vi "TestHarnessDPL-DetBoardOnly-DESKTOP-REOD41B.vi"() -> ()   [LabVIEW 2025]
uses:
  <vilib>/Analysis/6fits.llb/Curve Fitting Criteria.ctl
  <vilib>/Analysis/1siggen.llb/Ramp Pattern by Samples.vi
  <vilib>/Analysis/1siggen.llb/Ramp Pattern by Delta.vi
  <vilib>/Analysis/NI_AALBase.lvlib
  <userlib>/_OpenG.lib/time/time.llb/openg_time.lvlib
  instr.lib/Detector SCPI/Detector SCPI.lvlib
  instr.lib/Keithley 24XX/Keithley 24XX.lvlib
  instr.lib/Keithley 648X Series/Keithley 648X Series.lvlib
  <vilib>/Analysis/NI_AALPro.lvlib
panel:
  out "error out":errorcluster
  out "OpVsCurrent":cluster{"Ramp Pattern":dbl[], dbl[]}[](array[cluster])
  in  "Exit":bool
  in  "Measurement Mode":T1(tab)
  in  "DetectorData":T2(array[cluster]) {"DAC Offset" min=1 max=4095 step=1}
  in  "SPI Clock":i64=1000000
  in  "Oversample":i32=1 min=1 max=4096
  in  "Power":bool=TRUE
  in  "Detector VISA":refnum<visa-resource-name>="Detector_EGSE"
  out "Detector Resource":refnum<visa-resource-name>="COM4"
  out "Voltage (V)":dbl[](array[numeric])=[3.264, 0.0, 12.488, 12.77]
  out "Current (mA)":dbl[](array[numeric])=[0.0, 0.0, 21.6, -3.65]
  in  "ThrowAway":i32=100 min=1 max=10000
  out "Detector EGSE ID String":string="Aberystwyth University,Enfys Detector,#01,v0.5.0\r\n"
  in  "Current source":refnum<visa-resource-name>
  in  "Channel":i32 min=0 max=7
  in  "Collection":enum16{"Science", "Debug"}(ring)
  in  "Tolerance":dbl
  in  "Target Counts":i32 min=0 max=4095
  in  "Find Offset":bool
  out "Searching...":bool
  out "BoardTemperature":dbl
  in  "Tab Control":enum32{"Counts", "All Counts", "Temperature"}(tab)
  out "Counts":dbl(graph)=160.194
  out "All Counts":T3(graph)
  out "Temperature":dbl(graph)=160.194
  in  "ResetVDACstats":bool
  in  "Gain":u16(ring) items=["High", "Med", "Low"]
  in  "DAC Value":i32=2076 min=0 max=4095 step=1
  in  "Detector":u16(ring) items=["SWIR", "MWIR"]
  out "Peak-to-Peak (counts)":dbl=0.0026870000001508743 format="%^.4g"
  out "rms (counts) 2":dbl=-2.7284841053187847e-12 format="%^.4g"
  out "Mean Value (counts)":dbl
  out "Elapsed(uS)":i32
  out "size":i32
  in  "Pause":bool
  out "XY Graph":cluster{dbl[], "subarray":dbl[]}(graph)
  in  "Detector 3":u16(ring) items=["SWIR", "MWIR"]
  in  "Gain 3":u16(ring) items=["High", "Med", "Low"]
  in  "trig":dbl=8.0 min=0.0 max=50.0
  in  "DetectorDAC":i32=2076 min=0 max=4095 step=1
  in  "Abort":bool
  out "Output vs current":cluster{"Ramp Pattern":dbl[], dbl[]}[](graph)
  in  "ISweep":bool
  in  "NPoints":i32=10 min=10 max=10000 step=1
  in  "MaxCurrent":dbl=1e-11 min=1e-11 max=1e-06
  in  "MinCurrent":dbl=1e-12 min=-10.0 max=10.0
  in  "Detector 4":u16(ring) items=["SWIR", "MWIR"]
  in  "LogSweep":bool
  in  "Gain 4":u16(ring) items=["High", "Med", "Low"]
  out "slope (counts/nA)":dbl
  out "intercept":dbl
  out "residue":dbl
  out "Max Deviation (counts)":dbl
  in  "DAC":i32 min=0 max=4095 step=1
  in  "Modulation Steps":i32=2 min=2 max=1000 step=1
  in  "Modulation Max":dbl min=0.0 max=10.0
  in  "Modulation Min":dbl min=-10.0 max=10.0
  in  "SweepLight":bool
  in  "Detector 7":u16(ring) items=["SWIR", "MWIR"]
  out "Output vs Light":cluster{dbl[], dbl[]}[](graph)
  in  "Gain 2":u16(ring) items=["High", "Med", "Low"]
  in  "Abort 2":bool
  in  "SweepVDAC":bool
  in  "ISource":dbl min=-1e-06 max=1e-06
  in  "VDAC Step":i32=1 min=1 max=100
  in  "VDAC Max":i32 min=0 max=4095
  in  "VDAC Min":i32 min=0 max=4000
  in  "Detector 5":u16(ring) items=["SWIR", "MWIR"]
  out "VDAC Sweep":cluster{dbl[], dbl[]}[](graph)
  in  "Abort SweepVDAC":bool
  in  "Step":bool
  in  "Delay 1 (ms)":i32
  in  "Current 2":dbl
  in  "Current 1":dbl
  out "Step Response":cluster{dbl[], "subarray":dbl[]}(graph)
  in  "chan (0)":i32
  out "exit":bool=TRUE
  # "3.3V supply"
  # "Heater"
  # "+12V Supply"
  # "-12V Supply"
  # "Pause button will halt collection and display.\nThis allows graph to be printed etc."
  # "Burst mode is intended to examine behaviour of the ADC\n\nA burst of readings is recorded on the EGSE and then gathered here."
  # "Light source modulated by USB205L working as voltage source connected to MOD input of LD250C\nreference photodiode monitored by 6846 picoammeter"
  # "Set current to Current#1. Waits for Delay 1 to stabilise, then switches to current 2 and reads 1000 readings as fast as possible"
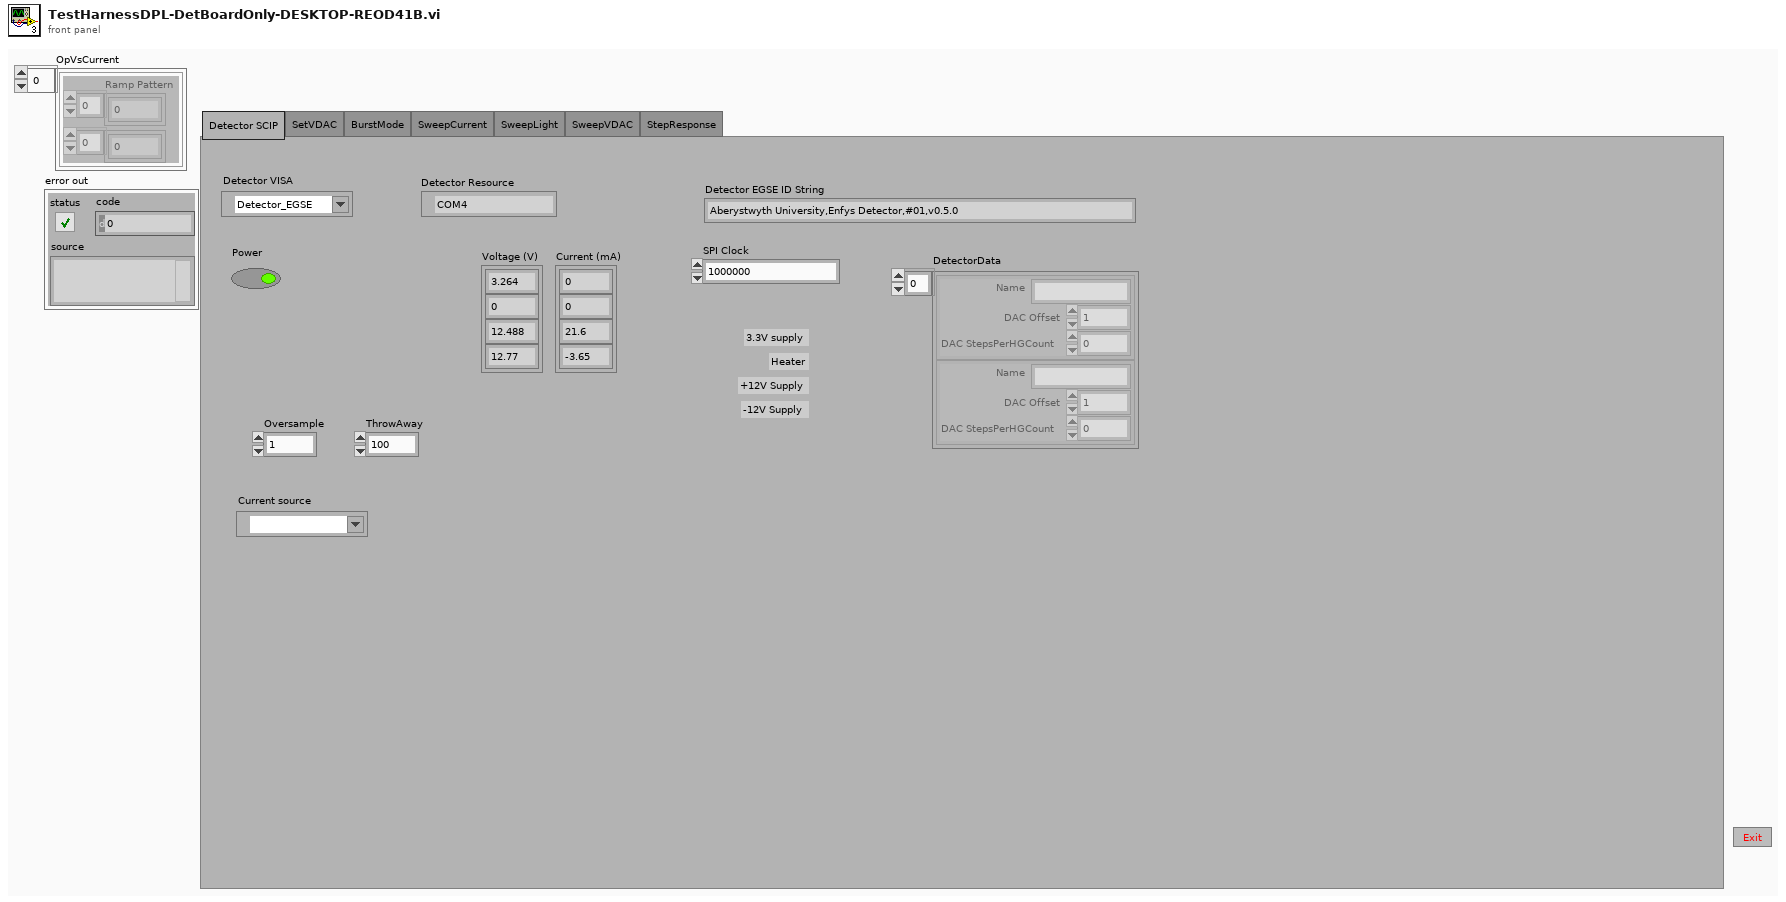
[diagram p1: front panel]
types:
  T1 = enum32{"Detector SCIP", "SetVDAC", "BurstMode", "SweepCurrent", "SweepLight", "SweepVDAC", "StepResponse"}
  T2 = cluster{"Name":string, "DAC Offset":i32, "DAC StepsPerHGCount":dbl}[]
  T3 = cluster{"subarray[0]":dbl, "subarray[1]":dbl, "subarray[2]":dbl, "subarray[3]":dbl, "subarray[4]":dbl, "subarray[5]":dbl, "subarray[6]":dbl, "subarray[7]":dbl, "subarray[8]":dbl}
  T4 = cluster{"Baud Rate":u32, "Parity":u16, "Data Bits":u16, "Stop Bits":u16, "Flow Control":u16}
  T5 = cluster{"Name":string, "DAC Offset":i32, "DAC StepsPerHGCount":dbl}
  T6 = typedef "NI_AALPro.lvlib/Curve Fitting Criteria.ctl" = u16
  T7 = typedef "LVPointDoubleTypeDef.ctl" = cluster{"Cursor X":dbl, "Cursor Y":dbl}
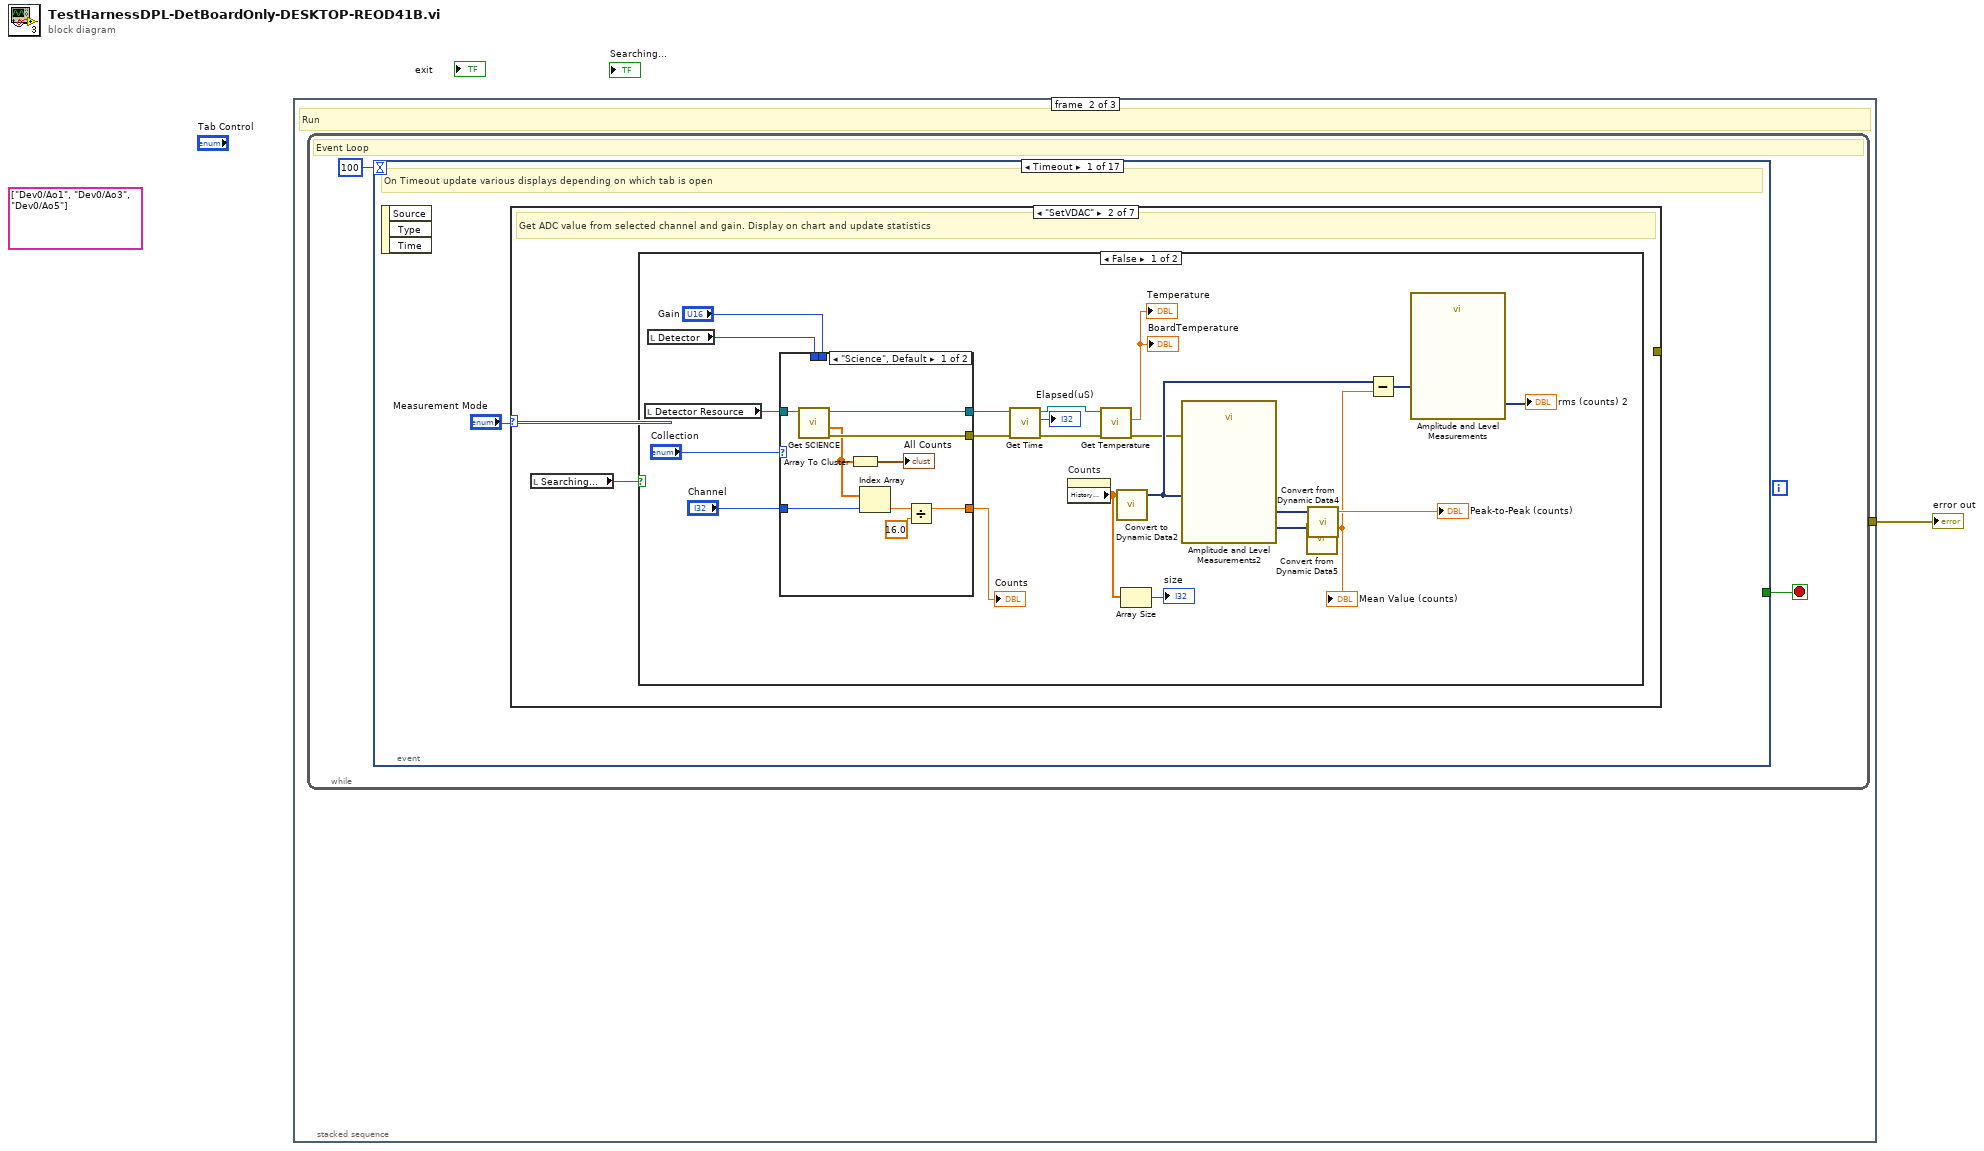
[diagram p0: block diagram]
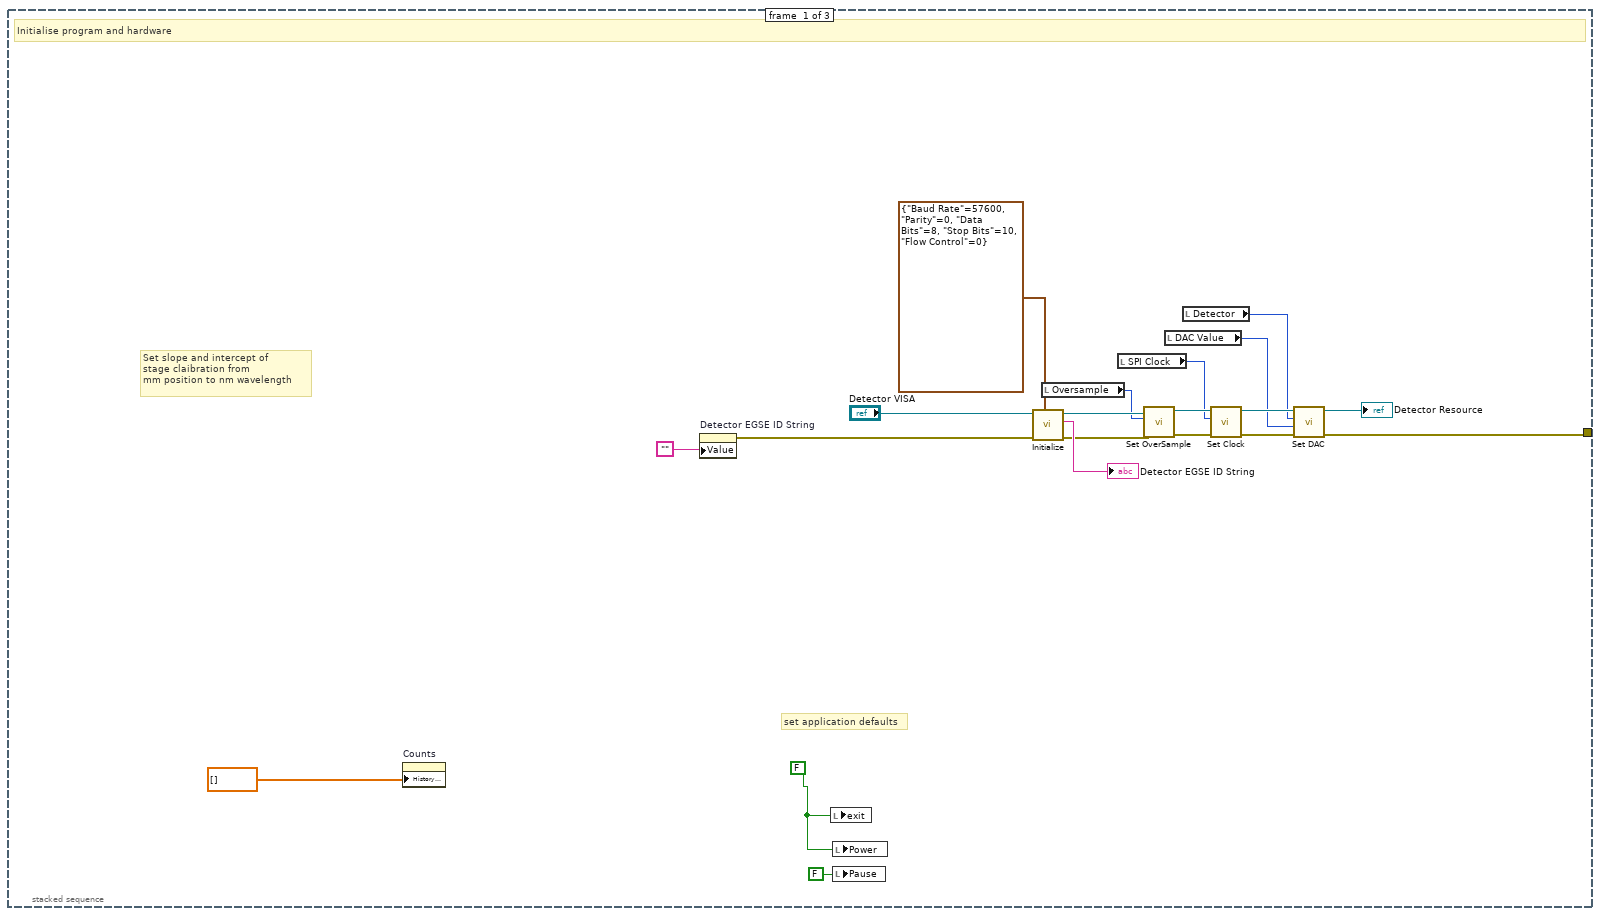
[diagram p2: hidden frame]
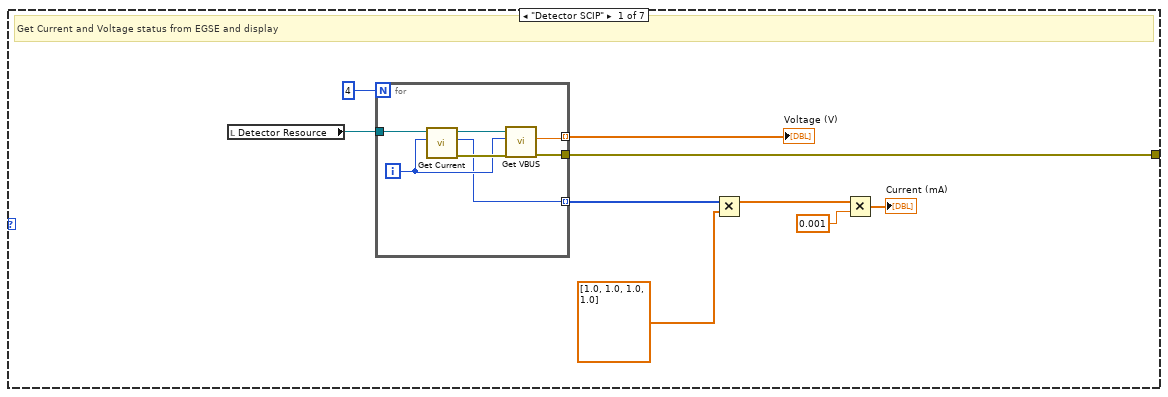
[diagram p3: hidden frame]
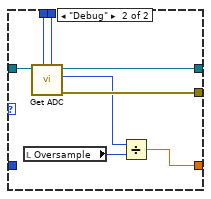
[diagram p4: hidden frame]
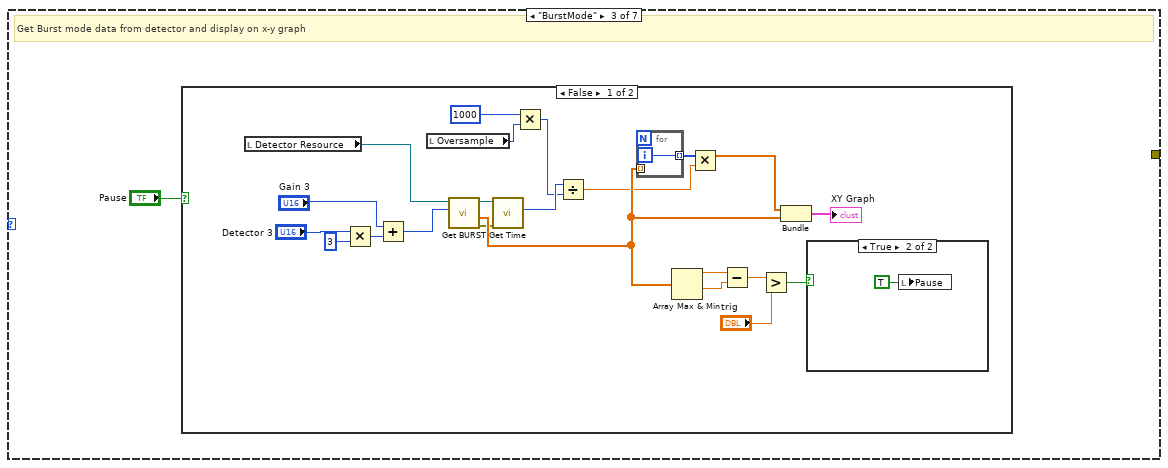
[diagram p6: hidden frame]
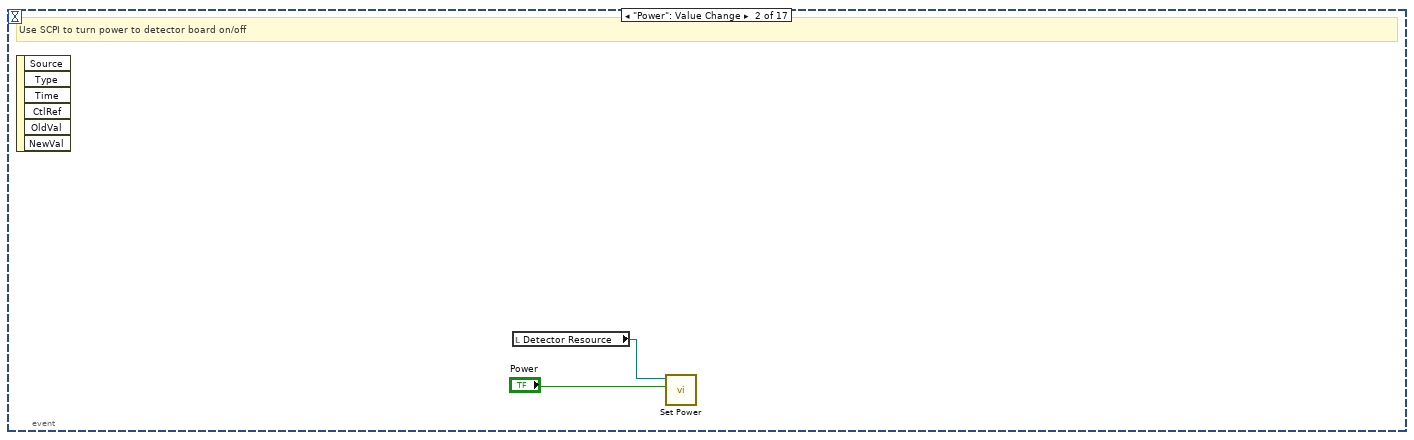
[diagram p13: hidden frame]
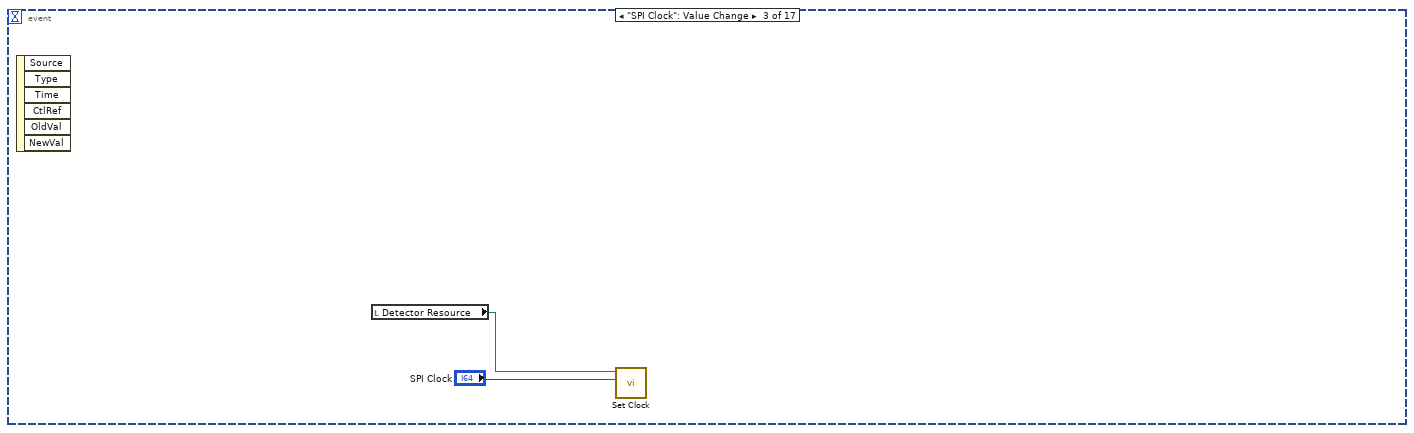
[diagram p14: hidden frame]
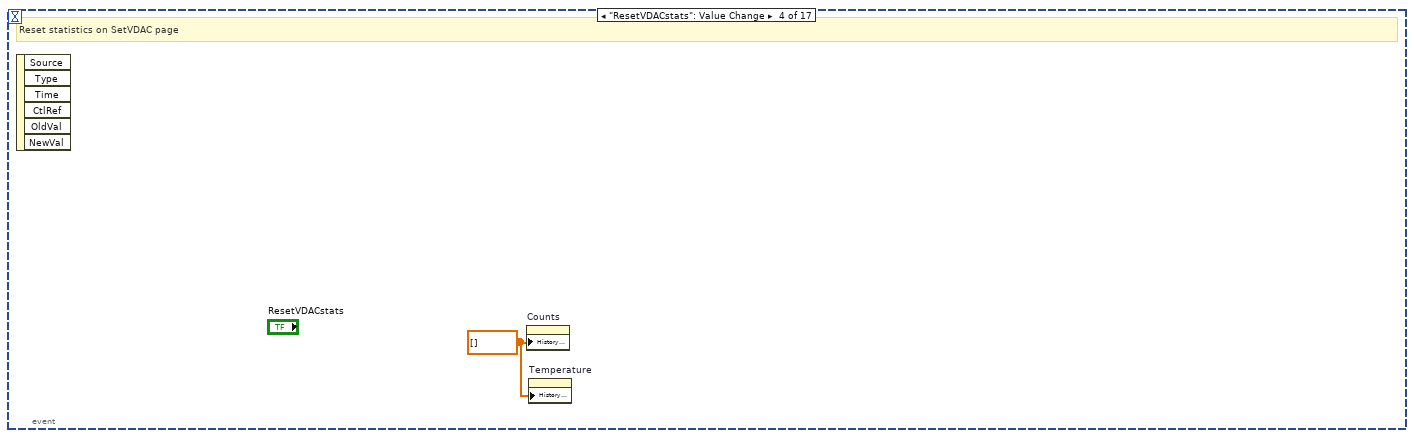
[diagram p15: hidden frame]
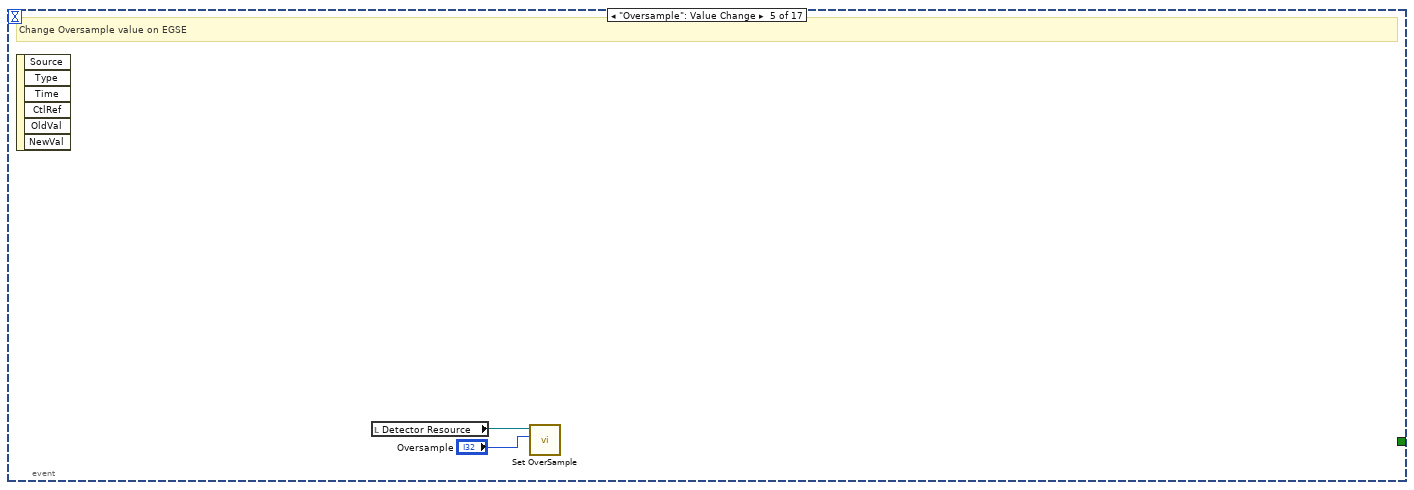
[diagram p16: hidden frame]
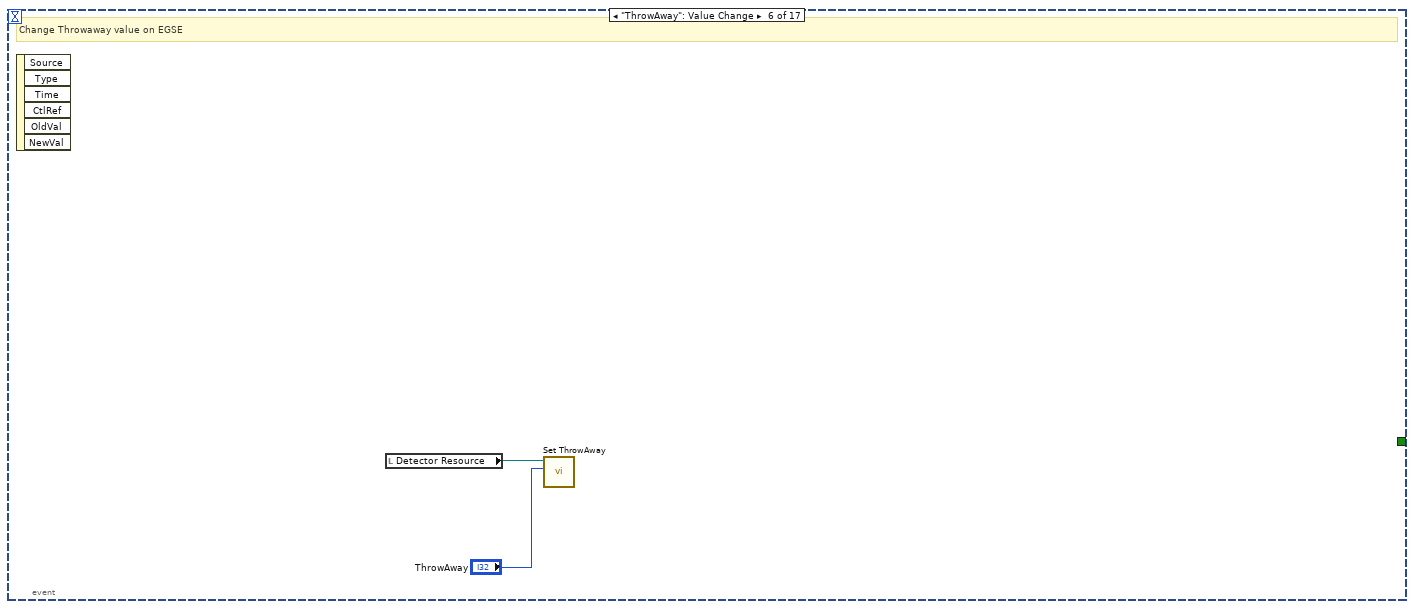
[diagram p17: hidden frame]
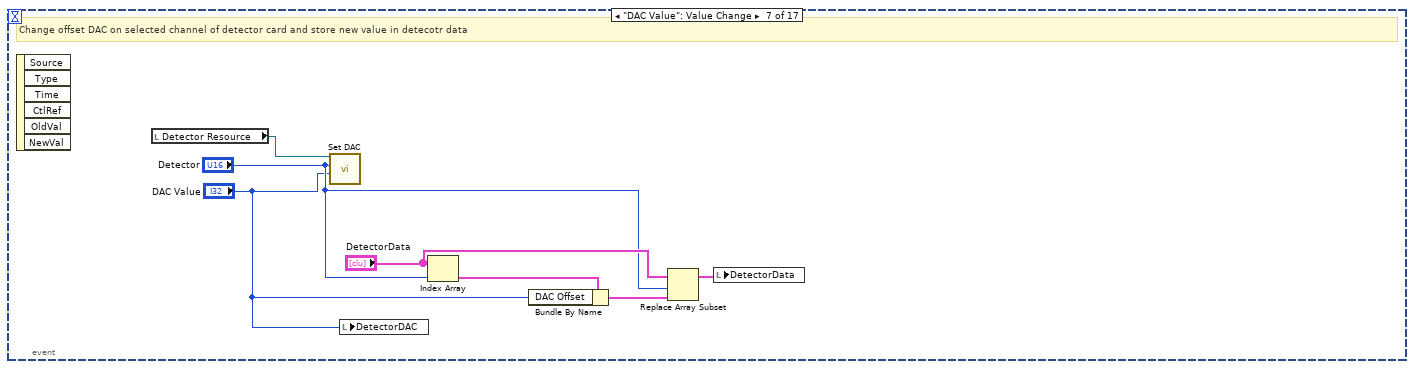
[diagram p18: hidden frame]
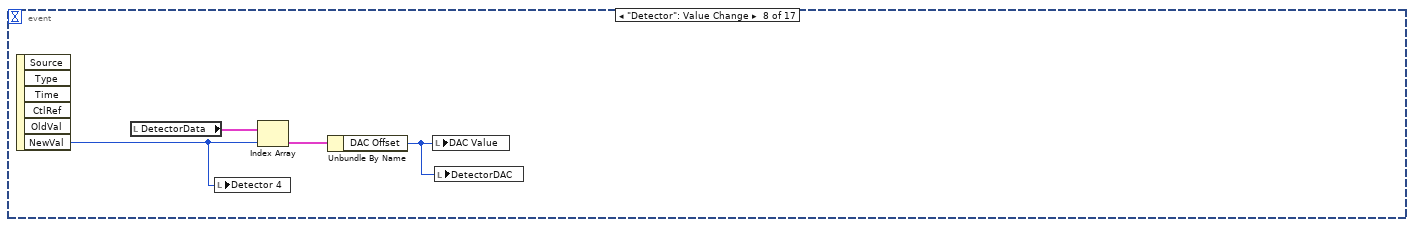
[diagram p19: hidden frame]
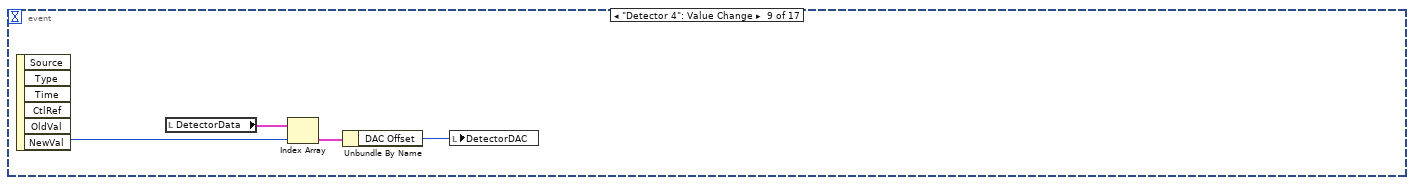
[diagram p20: hidden frame]
diagram:
  (unwired) string[] ["Dev0/Ao1", "Dev0/Ao3", "Dev0/Ao5"]
  n1 = stacked-sequence {
    tunnel: [w2 _ _] -> w1
    frame #0 {
      w20 = FALSE ("connected")
      # "Set slope and intercept of \nstage claibration from\nmm position to nm wavelength"
      # "set application defaults"
      # "Initialise program and hardware"
      n2 = property on="Counts" class="WFChart (strict)"("History Data"=dbl[] []) -> ()  [unwired: 2 in, 2 out]
      n3 = property on="Detector EGSE ID String" class="Str"("Value"="") -> (error out=w18:errorcluster)  [unwired: 2 in, 1 out]
      n4 = local write "exit"(w20) -> ()
      n5 = local write "Power"(w20) -> ()
      n6 = local write "Pause"(FALSE ("Pause")) -> ()
      n7 = call "Initialize.vi"("Serial Configuration"=T4 {"Baud Rate"=57600, "Parity"=0, "Data Bits"=8, "Stop Bits"=10, "Flow Control"=0}, "error in (no error)"=w18, "VISA resource name"="Detector VISA") -> ("error out"=w14:errorcluster, "ID String"=→"Detector EGSE ID String":string, "VISA resource name out"=w13:refnum<visa-resource-name>)  [unwired: 6 in]
      n8 = local read "Oversample"() -> (w12:i32)
      n9 = local read "SPI Clock"() -> (w7:i64)
      n10 = call "Set OverSample.vi"("error in (no error)"=w14, "oversample (0)"=w12, "VISA resource name"=w13) -> ("error out"=w11:errorcluster, "VISA resource name out"=w9:refnum<visa-resource-name>)  [unwired: 7 in]
      n11 = local read "DAC Value"() -> (w5:i32)
      n12 = local read "Detector"() -> (w6:u16)
      n13 = call "Set Clock.vi"("error in (no error)"=w11, "ClockSpeed"=w7, "VISA resource name"=w9) -> ("error out"=w10:errorcluster, "VISA resource name out"=w8:refnum<visa-resource-name>)  [unwired: 7 in]
      n14 = call "Set DAC.vi"("error in (no error)"=w10, "value (0)"=w5, "chan (0)"=w6, "VISA resource name"=w8) -> ("error out"=w2:errorcluster, "VISA resource name out"=→"Detector Resource":refnum<visa-resource-name>)  [unwired: 6 in]
    }
    frame #1 {
      # "Run"
      n15 = while {
        stop <- w22 stop-if-true
        # "Event Loop"
        n16 = event shown="[0] Timeout" {
          selector: _ -> [_ _ _ _ _ _ _ _ _ _ _ _ _ _ _ _ _]
          dyn-events: _ -> [_ _ _ _ _ _ _ _ _ _ _ _ _ _ _ _ _]
          timeout: 100 -> [_ _ _ _ _ _ _ _ _ _ _ _ _ _ _ _ _]
          tunnel: [_ _ _ _ _ _ _ _ _ _ _ _ _ _ _ "Exit" _] -> w22
          event Timeout {
            # "On Timeout update various displays depending on which tab is open"
            n17 = event-data() -> ()  [unwired: 1 in, 3 out]
            n18 = case shown="\"SetVDAC\"" "Measurement Mode" {
              tunnel: [w25 _ _ _ _ _ _] -> _
              frame "Detector SCIP" {
                # "Get Current and Voltage status from EGSE and display"
                n19 = local read "Detector Resource"() -> (w33:refnum<visa-resource-name>)
                n20 = for {
                  N: 4 -> [_]
                  tunnel: w33 -> [w40]
                  tunnel: [w36] -> w30 mode=indexing
                  tunnel: [w35] -> w31 mode=indexing
                  tunnel: [w34] -> w25
                  i -> [w37]
                  n21 = call "Get Current.vi"("chan (1)"=w37, "VISA resource name"=w40) -> ("error out"=w39:errorcluster, "output"=w36:i32, "VISA resource name out"=w38:refnum<visa-resource-name>)  [unwired: 7 in]
                  n22 = call "Get VBUS.vi"("error in (no error)"=w39, "chan (1)"=w37, "VISA resource name"=w38) -> ("error out"=w34:errorcluster, "output"=w35:dbl)  [unwired: 6 in, 1 out]
                }
                "Voltage (V)" <- w31
                n23 = Multiply(x=w30, y=dbl[] [1.0, 1.0, 1.0, 1.0]) -> (x*y=w27:dbl[])
                n24 = Multiply(x=w27, y=0.001) -> (x*y=→"Current (mA)":dbl[])
              }
              frame "SetVDAC" {
                # "Get ADC value from selected channel and gain. Display on chart and update statistics"
                n25 = local read "Searching..."() -> (w41:bool)
                n26 = case shown="False" w41 {
                  frame False {
                    n27 = local read "Detector Resource"() -> (w63:refnum<visa-resource-name>)
                    n28 = local read "Detector"() -> (w61:u16)
                    n29 = case shown="\"Science\", Default" "Collection" {
                      tunnel: w63 -> [w72 w80]
                      tunnel: "Gain" -> [_ w79]
                      tunnel: w61 -> [_ w78]
                      tunnel: [w71 w77] -> w60
                      tunnel: [w70 w76] -> w59
                      tunnel: [w65 w74] -> w43
                      tunnel: "Channel" -> [w69 _]
                      frame "Science", Default {
                        n30 = call "Get SCIENCE.vi"("VISA resource name"=w72) -> ("error out"=w70:errorcluster, "subarray"=w67:dbl[], "VISA resource name out"=w71:refnum<visa-resource-name>)  [unwired: 7 in, 1 out]
                        n31 = Array To Cluster(array=w67) -> (cluster=→"All Counts":T3)
                        n32 = Index Array(array=w67, index=w69) -> (element=w68:dbl)
                        n33 = Divide(x=w68, y=16.0) -> (x/y=w65:dbl)
                      }
                      frame "Debug" {
                        n34 = local read "Oversample"() -> (w75:i32)
                        n35 = call "Get ADC.vi"("Gain"=w79, "Detector"=w78, "VISA resource name"=w80) -> ("error out"=w76:errorcluster, "output"=w73:i32, "VISA resource name out"=w77:refnum<visa-resource-name>)  [unwired: 6 in]
                        n36 = Divide(x=w73, y=w75) -> (x/y=w74:dbl)
                      }
                    }
                    "Counts" <- w43
                    n37 = call "Get Time.vi"("error in (no error)"=w59, "VISA resource name"=w60) -> ("error out"=w47:errorcluster, "output"=→"Elapsed(uS)":i32, "VISA resource name out"=w45:refnum<visa-resource-name>)  [unwired: 7 in]
                    n38 = property on="Counts" class="WFChart (strict)"() -> ("History Data"=w50:dbl[])  [unwired: 2 in, 2 out]
                    n39 = call "Get Temperature.vi"("error in (no error)"=w47, "VISA resource name"=w45) -> ("error out"=w46:errorcluster, "output"=→"Temperature" →"BoardTemperature":dbl)  [unwired: 7 in, 1 out]
                    n40 = call "Convert to Dynamic Data2"("Array"=w50) -> ("Dynamic Data Type"=w51:dynamicdata)  [unwired: 3 in]
                    n41 = Array Size(array=w50) -> (size(s)=→"size":i32)
                    n42 = call "Amplitude and Level Measurements2"("Signals"=w51, "error in (no error)"=w46) -> ("Mean (DC)"=w53:dynamicdata, "Peak to Peak"=w56:dynamicdata)  [unwired: 10 in, 2 out]
                    n43 = call "Convert from Dynamic Data5"("Dynamic Data Type"=w53) -> ("Scalar"=w52:dbl)  [unwired: 3 in]
                    "Mean Value (counts)" <- w52
                    n44 = call "Convert from Dynamic Data4"("Dynamic Data Type"=w56) -> ("Scalar"=→"Peak-to-Peak (counts)":dbl)  [unwired: 3 in]
                    n45 = Subtract(x=w51, y=w52) -> (x-y=w54:dynamicdata)
                    n46 = call "Amplitude and Level Measurements"("Signals"=w54) -> ("RMS"=→"rms (counts) 2":dynamicdata)  [unwired: 11 in, 3 out]
                  }
                  frame True {
                  }
                }
              }
              frame "BurstMode" {
                # "Get Burst mode data from detector and display on x-y graph"
                n47 = case shown="False" "Pause" {
                  frame False {
                    n48 = local read "Detector Resource"() -> (w103:refnum<visa-resource-name>)
                    n49 = Multiply(x="Detector 3", y=u16 3) -> (x*y=w102:u16)
                    n50 = Add(x="Gain 3", y=w102) -> (x+y=w100:u16)
                    n51 = local read "Oversample"() -> (w87:i32)
                    n52 = call "Get BURST.vi"("chan (0)"=w100, "VISA resource name"=w103) -> ("error out"=w89:errorcluster, "subarray"=w95:dbl[], "VISA resource name out"=w88:refnum<visa-resource-name>)  [unwired: 6 in, 1 out]
                    n53 = call "Get Time.vi"("error in (no error)"=w89, "VISA resource name"=w88) -> ("output"=w86:i32)  [unwired: 7 in, 2 out]
                    n54 = Multiply(x=1000, y=w87) -> (x*y=w83:i32)
                    n55 = Divide(x=w86, y=w83) -> (x/y=w84:dbl)
                    n56 = for {
                      tunnel: w95 -> [_] mode=indexing
                      tunnel: [w105] -> w96 mode=indexing
                      i -> [w105]
                    }
                    n57 = Array Max & Min(array=w95) -> (max value=w94:dbl, min value=w93:dbl)  [unwired: 2 out]
                    n58 = Multiply(x=w96, y=w84) -> (x*y=w85:dbl[])
                    n59 = Subtract(x=w94, y=w93) -> (x-y=w92:dbl)
                    n60 = Greater?(x=w92, y="trig") -> (0:w90:bool)
                    n61 = Bundle(w85, "subarray"=w95) -> (→"XY Graph":cluster{dbl[], "subarray":dbl[]})  [unwired: 1 in]
                    n62 = case shown="True" w90 {
                      frame False {
                      }
                      frame True {
                        n63 = local write "Pause"(TRUE ("Pause")) -> ()
                      }
                    }
                  }
                  frame True {
                  }
                }
              }
              frame "SweepCurrent" {
              }
              frame "SweepVDAC" {
              }
              frame "StepResponse" {
              }
              frame "SweepLight" {
              }
            }
          }
          event "Power": Value Change {
            # "Use SCPI to turn power to detector board on/off"
            n64 = event-data() -> ()  [unwired: 1 in, 6 out]
            n65 = local read "Detector Resource"() -> (w107:refnum<visa-resource-name>)
            n66 = call "Set Power.vi"("Power (0)"="Power", "VISA resource name"=w107) -> ()  [unwired: 8 in, 2 out]
          }
          event "SPI Clock": Value Change {
            n67 = event-data() -> ()  [unwired: 1 in, 6 out]
            n68 = local read "Detector Resource"() -> (w109:refnum<visa-resource-name>)
            n69 = call "Set Clock.vi"("ClockSpeed"="SPI Clock", "VISA resource name"=w109) -> ()  [unwired: 8 in, 2 out]
          }
          event "ResetVDACstats": Value Change {
            w110 = dbl[] [] ("History Data")
            # "Reset statistics on SetVDAC page"
            n70 = event-data() -> ()  [unwired: 1 in, 6 out]
            n71 = property on="Counts" class="WFChart (strict)"("History Data"=w110) -> ()  [unwired: 2 in, 2 out]
            n72 = property on="Temperature" class="WFChart (strict)"("History Data"=w110) -> ()  [unwired: 2 in, 2 out]
          }
          event "Oversample": Value Change {
            # "Change Oversample value on EGSE"
            n73 = event-data() -> ()  [unwired: 1 in, 6 out]
            n74 = local read "Detector Resource"() -> (w112:refnum<visa-resource-name>)
            n75 = call "Set OverSample.vi"("oversample (0)"="Oversample", "VISA resource name"=w112) -> ()  [unwired: 8 in, 2 out]
          }
          event "ThrowAway": Value Change {
            # "Change Throwaway value on EGSE"
            n76 = event-data() -> ()  [unwired: 1 in, 6 out]
            n77 = local read "Detector Resource"() -> (w114:refnum<visa-resource-name>)
            n78 = call "Set ThrowAway.vi"("ThrowAway (0)"="ThrowAway", "VISA resource name"=w114) -> ()  [unwired: 8 in, 2 out]
          }
          event "DAC Value": Value Change {
            # "Change offset DAC on selected channel of detector card and store new value in detecotr data"
            n79 = event-data() -> ()  [unwired: 1 in, 6 out]
            n80 = local read "Detector Resource"() -> (w121:refnum<visa-resource-name>)
            n81 = call "Set DAC.vi"("value (0)"="DAC Value", "chan (0)"="Detector", "VISA resource name"=w121) -> ()  [unwired: 7 in, 2 out]
            n82 = local write "DetectorDAC"("DAC Value") -> ()
            n83 = Index Array(array="DetectorData", index="Detector") -> (element=w120:T5)
            n84 = Bundle By Name(cluster=w120, "DAC Offset"="DAC Value") -> (w117:T5)
            n85 = Replace Array Subset(array="DetectorData", new element=w117, index="Detector") -> (w116:T2)
            n86 = local write "DetectorData"(w116) -> ()
          }
          event "Detector": Value Change {
            n87 = event-data() -> ("NewVal"=w122:u16)  [unwired: 1 in, 5 out]
            n88 = local read "DetectorData"() -> (w125:T2)
            n89 = local write "Detector 4"(w122) -> ()
            n90 = Index Array(array=w125, index=w122) -> (element=w124:T5)
            n91 = Unbundle By Name(w124) -> ("DAC Offset"=w123:i32)
            n92 = local write "DAC Value"(w123) -> ()
            n93 = local write "DetectorDAC"(w123) -> ()
          }
          event "Detector 4": Value Change {
            n94 = event-data() -> ("NewVal"=w128:u16)  [unwired: 1 in, 5 out]
            n95 = local read "DetectorData"() -> (w129:T2)
            n96 = Index Array(array=w129, index=w128) -> (element=w127:T5)
            n97 = Unbundle By Name(w127) -> ("DAC Offset"=w126:i32)
            n98 = local write "DetectorDAC"(w126) -> ()
          }
          event "ISweep": Value Change {
            n99 = event-data() -> ()  [unwired: 1 in, 6 out]
            n100 = case shown="True" "ISweep" {
              frame False {
              }
              frame True {
                w136 = u16 50 items=["60 Hz"=60, "50 Hz or 400 Hz"=50] ("Power Line Frequency  (60 Hz)")
                w146 = u16 1 items=["Voltage", "Current"] ("Source Mode  (0: Voltage)")
                w155 = u16 1 items=["Volts", "Current", "Resistance"] ("Function (0: Volts)")
                w158 = u16 0 items=["Volts", "Current", "Resistance"] ("Function (0: Volts)")
                w162 = u16 1 items=["Voltage", "Current"] ("Source Mode  (0: Voltage)")
                w173 = dbl[] []
                # "wait 1000ms\nfor output to stabilise before clearing task"
                n101 = call "Initialize.vi"("ID Query (True)"=FALSE, "VISA resource name"=refnum<visa-resource-name> "B2901BL") -> ("error out"=w137:errorcluster, "VISA resource name out"=w140:refnum<visa-resource-name>)  [unwired: 8 in]
                n102 = call "Configure Power Line Frequency.vi"("error in (no error)"=w137, "Power Line Frequency  (60 Hz)"=w136, "VISA resource name"=w140) -> ("error out"=w138:errorcluster, "VISA resource name out"=w139:refnum<visa-resource-name>)  [unwired: 7 in]
                n103 = call "Configure Measurement.vi"("error in (no error)"=w138, "Enable Auto Range (T:Enable)"=TRUE, "Function (0: Volts)"=w158, "VISA resource name"=w139) -> ("error out"=w153:errorcluster, "VISA resource name out"=w154:refnum<visa-resource-name>)  [unwired: 6 in]
                n104 = call "Configure Measurement.vi"("error in (no error)"=w153, "Enable Auto Range (T:Enable)"=TRUE, "Function (0: Volts)"=w155, "VISA resource name"=w154) -> ("error out"=w135:errorcluster, "VISA resource name out"=w134:refnum<visa-resource-name>)  [unwired: 6 in]
                n105 = local read "Detector Resource"() -> (w180:refnum<visa-resource-name>)
                n106 = VISA Write(VISA resource name=w134, write buffer=":SOUR:CURR:RANGE 1e-4", error in (no error)=w135) -> (VISA resource name out=w133:refnum<visa-resource-name>, error out=w132:errorcluster)  [unwired: 1 out]
                n107 = case shown="False" "LogSweep" {
                  tunnel: "MaxCurrent" -> [w190 w194]
                  tunnel: "MinCurrent" -> [w189 w193]
                  tunnel: [w190 w192] -> w184
                  tunnel: [w189 w191] -> w183
                  frame False {
                  }
                  frame True {
                    n108 = Logarithm Base 10(1:w194) -> (0:w192:dbl)
                    n109 = Logarithm Base 10(1:w193) -> (0:w191:dbl)
                  }
                }
                n110 = call "Configure Output.vi"("Source Mode  (0: Voltage)"=w162, "error in (no error)"=w132, "Output Level (0)"=0.0, "VISA resource name"=w133) -> ("error out"=w161:errorcluster, "VISA resource name out"=w160:refnum<visa-resource-name>)  [unwired: 6 in]
                n111 = local read "Gain 4"() -> (w165:u16)
                n112 = call "Enable Output.vi"("error in (no error)"=w161, "Enable Output (T: Enable)"=TRUE ("Auto Output-Off (F: Disable)"), "VISA resource name"=w160) -> ("error out"=w151:errorcluster, "VISA resource name out"=w150:refnum<visa-resource-name>)  [unwired: 7 in]
                n113 = call "Set DAC.vi"("error in (no error)"=w151, "value (0)"="DetectorDAC", "chan (0)"="Detector 4", "VISA resource name"=w180) -> ("error out"=w175:errorcluster, "VISA resource name out"=w179:refnum<visa-resource-name>)  [unwired: 6 in]
                n114 = call-poly <vilib>:"Ramp Pattern.vi"("start"=w183, "end"=w184, "samples"="NPoints") -> ("Ramp Pattern"=w185:dbl[])  [unwired: 7 in, 1 out]
                n115 = local read "Oversample"() -> (w181:i32)
                n116 = property on="Gain" class="Ring (strict)"() -> (error out=w166:errorcluster, "Strings []"=w171:string[])  [unwired: 2 in, 1 out]
                n117 = call <userlib>:"Wait (ms)__ogtk.vi"("error in (no error)"=w175, "milliseconds to wait"=u32 1000) -> ("error out"=w176:errorcluster)  [unwired: 8 in, 1 out]
                n118 = case shown="False" "LogSweep" {
                  tunnel: w185 -> [w195 w197]
                  tunnel: [w195 w196] -> w182
                  frame False {
                  }
                  frame True {
                    n119 = Power Of 10(x=w197) -> (10^x=w196:dbl[])
                  }
                }
                n120 = Index Array(array=w171, index=w165) -> (element=w167:string)
                n121 = for {
                  tunnel: w176 -> [w211]
                  tunnel: w182 -> [w200] mode=indexing
                  tunnel: [w209] -> w141
                  shift-right: [w217] -> _
                  shift-left: w173 -> [w219]
                  tunnel: w182 -> [w204]
                  tunnel: w179 -> [w216]
                  tunnel: w181 -> [w213]
                  tunnel: "Detector 4" -> [w212]
                  tunnel: [w210] -> w142
                  tunnel: [w202] -> w172
                  tunnel: w173 -> [w203]
                  tunnel: w150 -> [w198]
                  stop <- "Abort" stop-if-true
                  w199 = u16 1 items=["Voltage", "Current"] ("Source Mode  (0: Voltage)")
                  n122 = call "Configure Output.vi"("Source Mode  (0: Voltage)"=w199, "error in (no error)"=w211, "Output Level (0)"=w200, "VISA resource name"=w198) -> ("error out"=w208:errorcluster, "VISA resource name out"=w210:refnum<visa-resource-name>)  [unwired: 6 in]
                  n123 = call <userlib>:"Wait Until Next ms Multiple__ogtk.vi"("error in (no error)"=w208, "milliseconds to wait"=u32 100) -> ("error out"=w207:errorcluster)  [unwired: 8 in, 1 out]
                  n124 = call "Get ADC.vi"("Gain"="Gain 4", "Detector"=w212, "error in (no error)"=w207, "VISA resource name"=w216) -> ("error out"=w209:errorcluster, "output"=w218:i32)  [unwired: 5 in, 1 out]
                  n125 = Divide(x=w218, y=w213) -> (x/y=w214:dbl)
                  n126 = Build Array (concatenate)(w219, w214) -> (w217:dbl[])
                  n127 = Bundle("Ramp Pattern"=w204, w217) -> (w205:cluster{"Ramp Pattern":dbl[], dbl[]})  [unwired: 1 in]
                  n128 = Bundle("Ramp Pattern"=w204, w203) -> (w201:cluster{"Ramp Pattern":dbl[], dbl[]})  [unwired: 1 in]
                  n129 = Build Array(w205, w201) -> (w202:cluster{"Ramp Pattern":dbl[], dbl[]}[])
                  "Output vs current" <- w202
                }
                "OpVsCurrent" <- w172
                n130 = property on="Output vs current" class="XYGraph (strict)"(error in=w166, "Active Plot"=u32 0) -> (error out=w168:errorcluster)  [unwired: 1 in, 1 out]
                n131 = property on="Output vs current" class="XYGraph (strict)"(error in=w168, "Plot.Plot Name"=w167) -> ()  [unwired: 1 in, 2 out]
                n132 = call "Configure Output.vi"("Source Mode  (0: Voltage)"=w146, "error in (no error)"=w141, "Output Level (0)"=0.0, "VISA resource name"=w142) -> ("error out"=w144:errorcluster, "VISA resource name out"=w143:refnum<visa-resource-name>)  [unwired: 6 in]
                n133 = call "Enable Output.vi"("error in (no error)"=w144, "Enable Output (T: Enable)"=FALSE ("Auto Output-Off (F: Disable)"), "VISA resource name"=w143) -> ("error out"=w148:errorcluster, "VISA resource name out"=w149:refnum<visa-resource-name>)  [unwired: 7 in]
                n134 = call "Close.vi"("error in (no error)"=w148, "VISA resource name"=w149) -> ()  [unwired: 9 in, 1 out]
              }
            }
          }
          event "Output vs current": Cursor Release {
            w239 = T6 0 items=["Least Square", "Least Absolute Residual", "Bisquare"] ("method")
            n135 = event-data() -> ()  [unwired: 1 in, 9 out]
            n136 = property on="Output vs current" class="XYGraph (strict)"("Active Cursor"=u32 0) -> (error out=w251:errorcluster)  [unwired: 2 in, 1 out]
            n137 = property on="Output vs current" class="XYGraph (strict)"(error in=w251) -> (error out=w248:errorcluster, "Cursor.Cursor Position"=w246:T7)  [unwired: 1 in, 1 out]
            n138 = Unbundle By Name(w246) -> ("Cursor X"=w234:dbl)
            n139 = local read "OpVsCurrent"() -> (w247:cluster{"Ramp Pattern":dbl[], dbl[]}[])
            n140 = property on="Output vs current" class="XYGraph (strict)"(error in=w248, "Active Cursor"=u32 1) -> (error out=w250:errorcluster)  [unwired: 1 in, 1 out]
            n141 = Index Array(array=w247) -> (element=w231:cluster{"Ramp Pattern":dbl[], dbl[]})  [unwired: 1 in]
            n142 = property on="Output vs current" class="XYGraph (strict)"(error in=w250) -> ("Cursor.Cursor Position"=w245:T7)  [unwired: 1 in, 2 out]
            n143 = Unbundle(w231) -> ("Ramp Pattern"=w244:dbl[], w242:dbl[])
            n144 = Unbundle By Name(w245) -> ("Cursor X"=w235:dbl)
            n145 = Max & Min(x=w235, y=w234) -> (max(x,y)=w232:dbl, min(x,y)=w233:dbl)
            n146 = Search 1D Array(1D array=w244, element=w233) -> (index of element=w241:i32)  [unwired: 1 in]
            n147 = local read "Output vs current"() -> (w229:cluster{"Ramp Pattern":dbl[], dbl[]}[])
            n148 = Search 1D Array(1D array=w244, element=w232) -> (index of element=w243:i32)  [unwired: 1 in]
            n149 = Subtract(x=w243, y=w241) -> (x-y=w240:i32)
            n150 = Array Subset(array=w242, index=w241, length=w240) -> (w224:dbl[])
            n151 = Array Subset(array=w244, index=w241, length=w240) -> (w230:dbl[])
            n152 = call <vilib>:"Linear Fit.vi"("Y"=w224, "X"=w230, "method"=w239) -> ("Best Linear Fit"=w225:dbl[], "slope"=→"slope (counts/nA)":dbl, "intercept"=→"intercept":dbl, "residue"=→"residue":dbl)  [unwired: 8 in, 1 out]
            n153 = Bundle(w230, "Best Linear Fit"=w225) -> (w227:cluster{dbl[], "Best Linear Fit":dbl[]})  [unwired: 1 in]
            n154 = Replace Array Subset(array=w229, new element=w227, index=1) -> (w226:cluster{"Ramp Pattern":dbl[], dbl[]}[])
            n155 = Subtract(x=w224, y=w225) -> (x-y=w223:dbl[])
            n156 = local write "Output vs current"(w226) -> ()
            n157 = Absolute Value(x=w223) -> (abs(x)=w222:dbl[])
            n158 = Array Max & Min(array=w222) -> (max value=→"Max Deviation (counts)":dbl)  [unwired: 3 out]
          }
          event "SweepLight": Value Change {
            n159 = event-data() -> ()  [unwired: 1 in, 6 out]
            n160 = case shown="True" "SweepLight" {
              frame False {
              }
              frame True {
                w270 = dbl[] []
                n161 = disable-structure shown="Disabled" {
                  disable-tunnel: [w280 _] -> w271
                  frame Disabled {
                    n162 = call "Keithley 648X Series SetupAcquisition.vi"("VISA resource name"=refnum<visa-resource-name> "Picoammeter") -> ("VISA resource name out"=w280:refnum<visa-resource-name>)  [unwired: 8 in, 1 out]
                  }
                  frame Enabled {
                  }
                }
                n163 = local read "Detector Resource"() -> (w278:refnum<visa-resource-name>)
                n164 = local read "Oversample"() -> (w279:i32)
                n165 = call-poly <vilib>:"Ramp Pattern.vi"("start"="Modulation Min", "end"="Modulation Max", "samples"="Modulation Steps") -> ("Ramp Pattern"=w274:dbl[])  [unwired: 7 in, 1 out]
                n166 = call "Set DAC.vi"("value (0)"="DAC", "chan (0)"="Detector 7", "VISA resource name"=w278) -> ("error out"=w269:errorcluster, "VISA resource name out"=w277:refnum<visa-resource-name>)  [unwired: 7 in]
                n167 = call "ULx Create Channel (AO-Voltage-Basic).vi"("maximum value"=5.0, "minimum value"=0.0, "physical channels"=refnum<k21> "Dev0/Ao0", "error in"=w269) -> ("task out"=w264:refnum<k24>, "error out"=w263:errorcluster)  [unwired: 10 in]
                n168 = call "ULx Write (Analog 1D DBL 1Chan 1Samp).vi"("task in"=w264, "data"="Modulation Min", "error in"=w263) -> ("task out"=w265:refnum<k24>, "error out"=w260:errorcluster)  [unwired: 10 in, 1 out]
                n169 = call <userlib>:"Wait (ms)__ogtk.vi"("error in (no error)"=w260, "milliseconds to wait"=u32 1000) -> ("error out"=w261:errorcluster)  [unwired: 8 in, 1 out]
                n170 = for {
                  tunnel: w261 -> [w310]
                  tunnel: [w309] -> w255
                  tunnel: [w291] -> w257
                  shift-right: [w304] -> _
                  shift-left: w270 -> [w306]
                  tunnel: w277 -> [w303]
                  shift-right: [w299] -> _
                  shift-left: w270 -> [w301]
                  shift-right: [w298] -> _
                  shift-left: w270 -> [w300]
                  tunnel: w279 -> [w293]
                  tunnel: "Detector 7" -> [w292]
                  tunnel: w274 -> [w284] mode=indexing
                  tunnel: w271 -> [w290]
                  shift-right: [w286] -> _
                  shift-left: w270 -> [w287]
                  tunnel: w265 -> [w285]
                  stop <- "Abort 2" stop-if-true
                  n171 = call "ULx Write (Analog 1D DBL 1Chan 1Samp).vi"("task in"=w285, "data"=w284, "error in"=w310) -> ("task out"=w309:refnum<k24>, "error out"=w308:errorcluster)  [unwired: 10 in, 1 out]
                  n172 = call "Get ADC.vi"("Gain"="Gain 2", "Detector"=w292, "error in (no error)"=w308, "VISA resource name"=w303) -> ("error out"=w302:errorcluster, "output"=w305:i32)  [unwired: 5 in, 1 out]
                  n173 = Divide(x=w305, y=w293) -> (x/y=w282:dbl)
                  n174 = Divide(x=w292, y=w293) -> ()  [unwired: 1 out]
                  n175 = Build Array (concatenate)(w301, w282) -> (w299:dbl[])
                  n176 = Build Array (concatenate)(w306, w282) -> (w304:dbl[])
                  n177 = Build Array (concatenate)(w300, w282) -> (w298:dbl[])
                  n178 = call "Measure Current.vi"("VISA resource name"=w290, "error in (no error)"=w302) -> ("Measurement"=w288:dbl, "error out"=w291:errorcluster)  [unwired: 11 in, 1 out]
                  n179 = Negate(x=w288) -> (-x=w283:dbl)
                  n180 = Build Array (concatenate)(w287, w283) -> (w286:dbl[])
                  n181 = Bundle(w286, w304) -> (w297:cluster{dbl[], dbl[]})  [unwired: 1 in]
                  n182 = Bundle(w286, w299) -> (w296:cluster{dbl[], dbl[]})  [unwired: 1 in]
                  n183 = Bundle(w286, w298) -> (w295:cluster{dbl[], dbl[]})  [unwired: 1 in]
                  n184 = Build Array(w297, w296, w295) -> (→"Output vs Light":cluster{dbl[], dbl[]}[])
                }
                n185 = call "ULx Write (Analog 1D DBL 1Chan 1Samp).vi"("task in"=w255, "data"=0.0, "error in"=w257) -> ("task out"=w256:refnum<k24>, "error out"=w258:errorcluster)  [unwired: 10 in, 1 out]
                n186 = call "ULx Clear Task.vi"("task in"=w256, "error in"=w258) -> ()  [unwired: 13 in, 1 out]
              }
            }
          }
          event "SweepVDAC": Value Change {
            n187 = event-data() -> ()  [unwired: 1 in, 6 out]
            n188 = case shown="True" "SweepVDAC" {
              frame False {
              }
              frame True {
                w324 = u16 1 items=["Voltage", "Current"] ("Source Mode  (0: Voltage)")
                w326 = dbl[] []
                w339 = u16 1 items=["Voltage", "Current"] ("Source Mode  (0: Voltage)")
                w343 = u16 1 items=["Volts", "Current", "Resistance"] ("Function (0: Volts)")
                w345 = u16 0 items=["Volts", "Current", "Resistance"] ("Function (0: Volts)")
                n189 = call "Initialize.vi"("ID Query (True)"=FALSE, "VISA resource name"="Current source") -> ("error out"=w331:errorcluster, "VISA resource name out"=w332:refnum<visa-resource-name>)  [unwired: 8 in]
                n190 = call "Configure Measurement.vi"("error in (no error)"=w331, "Enable Auto Range (T:Enable)"=TRUE, "Function (0: Volts)"=w345, "VISA resource name"=w332) -> ("error out"=w346:errorcluster, "VISA resource name out"=w347:refnum<visa-resource-name>)  [unwired: 6 in]
                n191 = call "Configure Measurement.vi"("Manual Range (1.0)"=1e-07, "error in (no error)"=w346, "Enable Auto Range (T:Enable)"=FALSE, "Function (0: Volts)"=w343, "VISA resource name"=w347) -> ("error out"=w341:errorcluster, "VISA resource name out"=w340:refnum<visa-resource-name>)  [unwired: 5 in]
                n192 = call-poly <vilib>:"Ramp Pattern.vi"("start"="VDAC Min", "end"="VDAC Max", "delta"="VDAC Step") -> ("Ramp Pattern"=w328:dbl[])  [unwired: 6 in, 2 out]
                n193 = local read "Oversample"() -> (w325:i32)
                n194 = local read "Detector Resource"() -> (w327:refnum<visa-resource-name>)
                n195 = call "Configure Output.vi"("Source Mode  (0: Voltage)"=w339, "error in (no error)"=w341, "Output Level (0)"="ISource", "VISA resource name"=w340) -> ("error out"=w338:errorcluster, "VISA resource name out"=w337:refnum<visa-resource-name>)  [unwired: 6 in]
                n196 = call "Enable Output.vi"("error in (no error)"=w338, "Enable Output (T: Enable)"=TRUE, "VISA resource name"=w337) -> ("error out"=w334:errorcluster, "VISA resource name out"=w335:refnum<visa-resource-name>)  [unwired: 7 in]
                n197 = for {
                  tunnel: w335 -> [w351]
                  tunnel: w334 -> [w382]
                  tunnel: w328 -> [w381] mode=indexing
                  tunnel: [w351] -> w323
                  tunnel: [w373] -> w321
                  shift-right: [w376] -> _
                  shift-left: w326 -> [w378]
                  tunnel: w328 -> [w364]
                  tunnel: w327 -> [w350]
                  shift-right: [w366] -> _
                  shift-left: w326 -> [w368]
                  shift-right: [w365] -> _
                  shift-left: w326 -> [w367]
                  tunnel: w325 -> [w354]
                  tunnel: "Detector 5" -> [w352]
                  stop <- "Abort SweepVDAC" stop-if-true
                  w369 = u16 2 items=["High", "Med", "Low"] ("Gain")
                  w370 = u16 1 items=["High", "Med", "Low"] ("Gain")
                  w379 = u16 0 items=["High", "Med", "Low"] ("Gain")
                  n198 = call "Set DAC.vi"("error in (no error)"=w382, "value (0)"=w381, "chan (0)"=w352, "VISA resource name"=w350) -> ("error out"=w380:errorcluster, "VISA resource name out"=w349:refnum<visa-resource-name>)  [unwired: 6 in]
                  n199 = call "Get ADC.vi"("Gain"=w379, "Detector"=w352, "error in (no error)"=w380, "VISA resource name"=w349) -> ("error out"=w375:errorcluster, "output"=w377:i32, "VISA resource name out"=w372:refnum<visa-resource-name>)  [unwired: 5 in]
                  n200 = Divide(x=w377, y=w354) -> (x/y=w358:dbl)
                  n201 = call "Get ADC.vi"("Gain"=w370, "Detector"=w352, "error in (no error)"=w375, "VISA resource name"=w372) -> ("error out"=w374:errorcluster, "output"=w357:i32, "VISA resource name out"=w371:refnum<visa-resource-name>)  [unwired: 5 in]
                  n202 = Divide(x=w357, y=w354) -> (x/y=w356:dbl)
                  n203 = call "Get ADC.vi"("Gain"=w369, "Detector"=w352, "error in (no error)"=w374, "VISA resource name"=w371) -> ("error out"=w373:errorcluster, "output"=w353:i32)  [unwired: 5 in, 1 out]
                  n204 = Divide(x=w353, y=w354) -> (x/y=w355:dbl)
                  n205 = Build Array (concatenate)(w368, w356) -> (w366:dbl[])
                  n206 = Build Array (concatenate)(w378, w358) -> (w376:dbl[])
                  n207 = Build Array (concatenate)(w367, w355) -> (w365:dbl[])
                  n208 = Bundle("Ramp Pattern"=w364, w376) -> (w363:cluster{"Ramp Pattern":dbl[], dbl[]})  [unwired: 1 in]
                  n209 = Bundle("Ramp Pattern"=w364, w366) -> (w362:cluster{"Ramp Pattern":dbl[], dbl[]})  [unwired: 1 in]
                  n210 = Bundle("Ramp Pattern"=w364, w365) -> (w361:cluster{"Ramp Pattern":dbl[], dbl[]})  [unwired: 1 in]
                  n211 = Build Array(w363, w362, w361) -> (→"VDAC Sweep":cluster{"Ramp Pattern":dbl[], dbl[]}[])
                }
                n212 = call "Configure Output.vi"("Source Mode  (0: Voltage)"=w324, "error in (no error)"=w321, "Output Level (0)"=0.0, "VISA resource name"=w323) -> ("error out"=w320:errorcluster, "VISA resource name out"=w322:refnum<visa-resource-name>)  [unwired: 6 in]
                n213 = call "Enable Output.vi"("error in (no error)"=w320, "Enable Output (T: Enable)"=FALSE, "VISA resource name"=w322) -> ("error out"=w330:errorcluster, "VISA resource name out"=w329:refnum<visa-resource-name>)  [unwired: 7 in]
                n214 = call "Close.vi"("error in (no error)"=w330, "VISA resource name"=w329) -> ()  [unwired: 9 in, 1 out]
              }
            }
          }
          event "Step": Value Change {
            n215 = event-data() -> ()  [unwired: 1 in, 6 out]
            n216 = case shown="True" "Step" {
              frame False {
              }
              frame True {
                w395 = 1000 ("oversample (0)")
                w407 = u16 1 items=["Voltage", "Current"] ("Source Mode  (0: Voltage)")
                w411 = u16 1 items=["Voltage", "Current"] ("Source Mode  (0: Voltage)")
                w414 = u16 1 items=["Volts", "Current", "Resistance"] ("Function (0: Volts)")
                w417 = u16 0 items=["Volts", "Current", "Resistance"] ("Function (0: Volts)")
                n217 = local read "Detector Resource"() -> (w391:refnum<visa-resource-name>)
                n218 = property on="Oversample" class="DigNum (strict)"() -> (error out=w403:errorcluster, "Value"=w386:i32)  [unwired: 2 in, 1 out]
                n219 = call "Set OverSample.vi"("error in (no error)"=w403, "oversample (0)"=w395, "VISA resource name"=w391) -> ("error out"=w404:errorcluster)  [unwired: 7 in, 1 out]
                n220 = local read "Current source"() -> (w384:refnum<visa-resource-name>)
                n221 = call "Initialize.vi"("error in (no error)"=w404, "ID Query (True)"=FALSE, "VISA resource name"=w384) -> ("error out"=w427:errorcluster, "VISA resource name out"=w426:refnum<visa-resource-name>)  [unwired: 7 in]
                n222 = call "Configure Measurement.vi"("error in (no error)"=w427, "Enable Auto Range (T:Enable)"=TRUE, "Function (0: Volts)"=w417, "VISA resource name"=w426) -> ("error out"=w421:errorcluster, "VISA resource name out"=w420:refnum<visa-resource-name>)  [unwired: 6 in]
                n223 = call "Configure Measurement.vi"("Manual Range (1.0)"=1e-07, "error in (no error)"=w421, "Enable Auto Range (T:Enable)"=FALSE, "Function (0: Volts)"=w414, "VISA resource name"=w420) -> ("error out"=w422:errorcluster, "VISA resource name out"=w423:refnum<visa-resource-name>)  [unwired: 5 in]
                n224 = call "Configure Output.vi"("Source Mode  (0: Voltage)"=w411, "error in (no error)"=w422, "Output Level (0)"="Current 1", "VISA resource name"=w423) -> ("error out"=w424:errorcluster, "VISA resource name out"=w425:refnum<visa-resource-name>)  [unwired: 6 in]
                n225 = call "Enable Output.vi"("error in (no error)"=w424, "Enable Output (T: Enable)"=TRUE, "VISA resource name"=w425) -> ("error out"=w410:errorcluster, "VISA resource name out"=w406:refnum<visa-resource-name>)  [unwired: 7 in]
                n226 = call <userlib>:"Wait (ms)__ogtk.vi"("error in (no error)"=w410, "milliseconds to wait"="Delay 1 (ms)") -> ("error out"=w408:errorcluster)  [unwired: 8 in, 1 out]
                n227 = call "Configure Output.vi"("Source Mode  (0: Voltage)"=w407, "error in (no error)"=w408, "Output Level (0)"="Current 2", "VISA resource name"=w406) -> ("error out"=w402:errorcluster, "VISA resource name out"=w388:refnum<visa-resource-name>)  [unwired: 6 in]
                n228 = call "Get BURST.vi"("error in (no error)"=w402, "chan (0)"="chan (0)", "VISA resource name"=w391) -> ("error out"=w400:errorcluster, "subarray"=w393:dbl[], "VISA resource name out"=w399:refnum<visa-resource-name>)  [unwired: 5 in, 1 out]
                n229 = for {
                  tunnel: w393 -> [_] mode=indexing
                  tunnel: [w428] -> w398 mode=indexing
                  i -> [w428]
                }
                n230 = call "Get Time.vi"("error in (no error)"=w400, "VISA resource name"=w399) -> ("error out"=w389:errorcluster, "output"=w397:i32, "VISA resource name out"=w385:refnum<visa-resource-name>)  [unwired: 7 in]
                n231 = Divide(x=w397, y=w395) -> (x/y=w396:dbl)
                n232 = Multiply(x=w396, y=w398) -> (x*y=w394:dbl[])
                n233 = Bundle(w394, "subarray"=w393) -> (→"Step Response":cluster{dbl[], "subarray":dbl[]})  [unwired: 1 in]
                n234 = call "Enable Output.vi"("error in (no error)"=w389, "Enable Output (T: Enable)"=TRUE, "VISA resource name"=w388) -> ("error out"=w387:errorcluster)  [unwired: 7 in, 1 out]
                n235 = call "Set OverSample.vi"("error in (no error)"=w387, "oversample (0)"=w386, "VISA resource name"=w385) -> ()  [unwired: 7 in, 2 out]
              }
            }
          }
          event "Find Offset": Value Change {
            n236 = event-data() -> ()  [unwired: 1 in, 6 out]
            n237 = property on="Searching..." class="Bool (strict)"("Value"=TRUE ("Searching...")) -> (error out=w433:errorcluster)  [unwired: 2 in, 1 out]
            n238 = while {
              shift-right: [w438] -> _
              shift-left: 4095 -> [w443]
              shift-right: [w441] -> _
              shift-left: 1 -> [w442]
              tunnel: w433 -> [w439]
              tunnel: [w437] -> w430
              stop <- w440 stop-if-true
              n239 = Subtract(x=w443, y=w442) -> (x-y=w445:i32)
              n240 = Absolute Value(x=w445) -> (abs(x)=w436:i32)
              n241 = Less Or Equal?(x=w436, y=1) -> (x <= y?=w444:bool)
              n242 = case shown="False" w444 {
                tunnel: w443 -> [w452 w486]
                tunnel: w442 -> [w451 w488]
                tunnel: [w450 w488] -> w441
                tunnel: [w454 TRUE] -> w440
                tunnel: w439 -> [w467 _]
                tunnel: [w448 w486] -> w438
                tunnel: [w447 _] -> w437
                frame False {
                  w461 = u16 0 items=["High", "Med", "Low"] ("Gain")
                  # "Not there yet."
                  n243 = local read "Detector Resource"() -> (w468:refnum<visa-resource-name>)
                  n244 = Add(x=w452, y=w451) -> (x+y=w470:i32)
                  n245 = Quotient & Remainder(x=w470, y=2) -> (floor(x/y)=w453:i32)  [unwired: 1 out]
                  n246 = local read "Detector"() -> (w462:u16)
                  n247 = local write "DAC Value"(w453) -> ()
                  n248 = call "Set DAC.vi"("error in (no error)"=w467, "value (0)"=w453, "chan (0)"=w462, "VISA resource name"=w468) -> ("error out"=w466:errorcluster, "VISA resource name out"=w463:refnum<visa-resource-name>)  [unwired: 6 in]
                  n249 = local read "Oversample"() -> (w460:i32)
                  n250 = call <userlib>:"Wait (ms)__ogtk.vi"("error in (no error)"=w466, "milliseconds to wait"=u32 5) -> ("error out"=w464:errorcluster)  [unwired: 8 in, 1 out]
                  n251 = call "Get ADC.vi"("Gain"=w461, "Detector"=w462, "error in (no error)"=w464, "VISA resource name"=w463) -> ("error out"=w447:errorcluster, "output"=w459:i32)  [unwired: 5 in, 1 out]
                  n252 = Divide(x=w459, y=w460) -> (x/y=w446:dbl)
                  n253 = Subtract(x=w446, y="Target Counts") -> (x-y=w449:dbl)
                  n254 = local write "Counts"(w446) -> ()
                  n255 = Absolute Value(x=w449) -> (abs(x)=w457:dbl)
                  n256 = Less?(x=w457, y="Tolerance") -> (x < y?=w455:bool)
                  n257 = case shown="True" w455 {
                    tunnel: [FALSE TRUE] -> w454
                    tunnel: w453 -> [w474 w484]
                    tunnel: w452 -> [w475 w483]
                    tunnel: w451 -> [w473 _]
                    tunnel: [w471 w484] -> w450
                    tunnel: w449 -> [w477 _]
                    tunnel: [w472 w483] -> w448
                    frame False {
                      # "Not there, so examine difference\nbetween target and reading"
                      n258 = Greater Than 0?(x=w477) -> (x > 0?=w476:bool)
                      n259 = case shown="True" w476 {
                        tunnel: w475 -> [_ w482]
                        tunnel: w474 -> [w480 w481]
                        tunnel: w473 -> [w479 _]
                        tunnel: [w480 w482] -> w472
                        tunnel: [w479 w481] -> w471
                        frame False {
                          # "Reading is below target, so next DAC vaue will be below midpoint"
                        }
                        frame True {
                          # "If reading is above target, then next DAC value will be above mid"
                        }
                      }
                    }
                    frame True {
                      # "Within tolerance, so finish"
                    }
                  }
                }
                frame True {
                  # "DAC Values identical so finish"
                }
              }
            }
            n260 = property on="Searching..." class="Bool (strict)"(error in=w430, "Value"=FALSE ("Searching...")) -> ()  [unwired: 1 in, 2 out]
          }
          event "Exit": Value Change {
            # "If stage is connected, go to reference position and then exit"
            n261 = event-data() -> ()  [unwired: 1 in, 6 out]
          }
          event Panel Close? {
            # "Discard \"Panel Close?\" event\n\nto leave program through\n graceful route"
            # "NOTE:\nMake sure not to use the red \"Abort Execution\" button in the\nLabVIEW menu to abort the application execution.\nDoing so will not close the device connection with the consequence that\na re-open after the next application start will fail."
            # "\"Panel Close\" (\"X\") was clicked by the user:\nWe discard the close command and set an \"exit\" flag. This gives us the change to proper disconnect the device and clean up the application before closing the window."
            # "Trap \"Panel Close\" instruction and exit program gracefully"
            n262 = event-data() -> ()  [unwired: 1 in, 4 out]
            n263 = local write "exit"(TRUE ("exit")) -> ()
            n264 = event-data("Discard?"=TRUE) -> ()  [unwired: 1 in, 1 out]
          }
        }
      }
    }
    frame #2 {
      # "Also power off and close detector SCPI EGSE"
      # "Cleanup and Shutdown"
      n265 = local read "Detector Resource"() -> (w496:refnum<visa-resource-name>)
      n266 = call "Set Power.vi"("Power (0)"=FALSE, "VISA resource name"=w496) -> ("error out"=w493:errorcluster, "VISA resource name out"=w497:refnum<visa-resource-name>)  [unwired: 8 in]
      n267 = property on="Power" class="Bool (strict)"(error in=w493, "Value"=FALSE ("Power")) -> (error out=w494:errorcluster)  [unwired: 1 in, 1 out]
      n268 = call "Close.vi"("error in (no error)"=w494, "VISA resource name"=w497) -> ()  [unwired: 9 in, 1 out]
    }
  }
  "error out" <- w1
